vi "Config HW Set.vi"(6 "Send Cmd Timout(ms)":u32=300, 7 "CANcoder Ref":T1, 8 "Error":errorcluster, 9 "HW Config":T7={"ExtendHW Ver"=0, "CAN"={"ID"=0, "Bus"=""}, "Output"={"Type"=enum."Counter-Clockwise", "Neutral"=enum."EEPROMSetting", "Max"={"FWD"=0.0, "REV"=-1.0}, "Min"={"FWD"=0.0, "REV"=0.0}, "OL Ramp Rate (S)"=0.0, "Dead Band"=0.0, "CL Ramp Rate (S)"=0.0}, "CL"={"Gains"={"P"=1.0, "I"=0.01, "D"=0.0, "F"=0.0}, "Error Allowed"=0.0, "I Zone"=0.0, "Peak Out 0-1"=10000.0, "Max I Accu"=-1000.0}, "MM"={"Cruise Velocity"=5000, "Acceleration"=5000}, "TravelLimits"={"Hard"={"FWD Switch Normal"=enum."Normally Open", "FWD On will Zero Encoder "=FALSE, "REV Switch Normal"=enum."Normally Open", "REV On will Zero Encoder "=FALSE}, "Soft"={"FWD"={"Enable"=FALSE, "Counts"=0}, "REV"={"Enable"=FALSE, "Counts"=0}}}, "StatorLimit"={"Enable"=FALSE, "Current Limit"=0.0, "Threshold Current"=0.0, "Threshold Time"=0.0}, "Cancoder"={"ID"=0, "CW(t) CCW(f)"=TRUE, "Zero Offset"=0.0}} {"TravelLimits"."Soft"."REV"."Counts" format="%#.0f"; "TravelLimits"."Soft"."FWD"."Counts" format="%#.0f"; "Output"."Min"."REV" format="%.2f"; "Output"."Min"."FWD" format="%.2f"; "Output"."Max"."REV" format="%.2f"; "Output"."Max"."FWD" format="%.2f"; "CL"."Gains"."F" format="%#.8f"; "CL"."Gains"."D" format="%#.8f"; "CL"."Gains"."I" format="%#.8f"; "CL"."Gains"."P" format="%#.8f"}, 10 "Max # Of Tries":i32, 11 "DevRef":T2={"DeviceStatus"={"status"=FALSE, "code"=0, "source"=""}, "Type"=enum."PWM", "PWM"={"PWM Channel"=enum."Invalid", "DeadBand"={"Name"="", "maxPositivePwm"=0, "minPositivePwm"=0, "centerPwm"=0, "maxNegativePwm"=0, "minNegativePwm"=0, "angularRange"=0}}, "CAN"={"Device Number"=0, "SetOutput VI Ref"=variant, "GetOutput VI Ref"=variant, "Enable VI Ref"=variant, "Disable VI Ref"=variant, "Data"=variant}, "Invert"=FALSE, "DIO PWM"={"PWM \"Enable\" Channel"=enum."Invalid", "DIOChannel"=enum."Invalid", "PWM Rate"=0.0}}) -> (0 "Error Out":errorcluster, 3 "DevRef Out Out":T2, 5 "CANcoder Ref Out":T1)   [LabVIEW 2023, in "2024 AdPivotArm_ACT.lvlib"]
uses:
  2024 AdPivotArm_ACT.lvlib
  Shared Code/TypeDefs/Cluster_Extend_Config HW Values.ctl
  Shared Code/TypeDefs/Cluser_CAN Data.ctl
  Shared Code/TypeDefs/Cluster_Config FX Motor Output.ctl
  <vilib>/Rock Robotics/WPI/ThirdParty/Phoenix-LabVIEW/Motor Controller/Controls/CTRE_Phoenix_MotorControl_TalonFXInvertType.ctl
  <vilib>/Rock Robotics/WPI/ThirdParty/Phoenix-LabVIEW/Motor Controller/Controls/CTRE_Phoenix_MotorControl_NeutralMode.ctl
  Shared Code/TypeDefs/Cluster_FWD  REV Values.ctl
  Shared Code/TypeDefs/Cluster_FX SLOT PID Config.ctl
  Shared Code/TypeDefs/Cluster_PID Gains.ctl
  Shared Code/TypeDefs/Cluster_FX Motion Magic Parameters.ctl
  Shared Code/TypeDefs/Cluser_FX Config_Limit Travel.ctl
  Shared Code/TypeDefs/Cluser_Hard Limits.ctl
  <vilib>/Rock Robotics/WPI/ThirdParty/Phoenix-LabVIEW/Motor Controller/Controls/CTRE_Phoenix_MotorControl_LimitSwitchNormal.ctl
  Shared Code/TypeDefs/Cluser_Config_Soft Limits.ctl
  Shared Code/TypeDefs/Cluser_Enable-Value I32.ctl
  Shared Code/TypeDefs/Cluser_FX Config_Current Limits.ctl
  Shared Code/TypeDefs/Cluster_Cancoder_Config Data.ctl
  <vilib>/Rock Robotics/WPI/MotorControl/WPI_MotorControlDeviceRef.ctl
  <vilib>/Rock Robotics/WPI/MotorControl/WPI_MotorControlType.ctl
  <vilib>/Rock Robotics/SystemInterfaces/DIO/FPGA_DIOPWMChannel.ctl
  <vilib>/Rock Robotics/WPI/PWM/WPI_PWMDeadband.ctl
  <vilib>/Rock Robotics/SystemInterfaces/DIO/FPGA_DIOChannel.ctl
  <vilib>/Rock Robotics/WPI/ThirdParty/Phoenix-LabVIEW/CANCoder/Controls/CTRE_Phoenix_CANcoder_DeviceRef.ctl
  Shared Code/TypeDefs/Cluster_Config Motor Output.ctl
  Shared Code/TypeDefs/Cluster_PID Config.ctl
  Shared Code/TypeDefs/Cluster_High-Low.ctl
  Shared Code/TypeDefs/Cluster_Motion Magic Parameters.ctl
  Shared Code/TypeDefs/Cluster_Config_Cancoder Data.ctl
panel:
  # "Tune Output\nto 1023 Max"
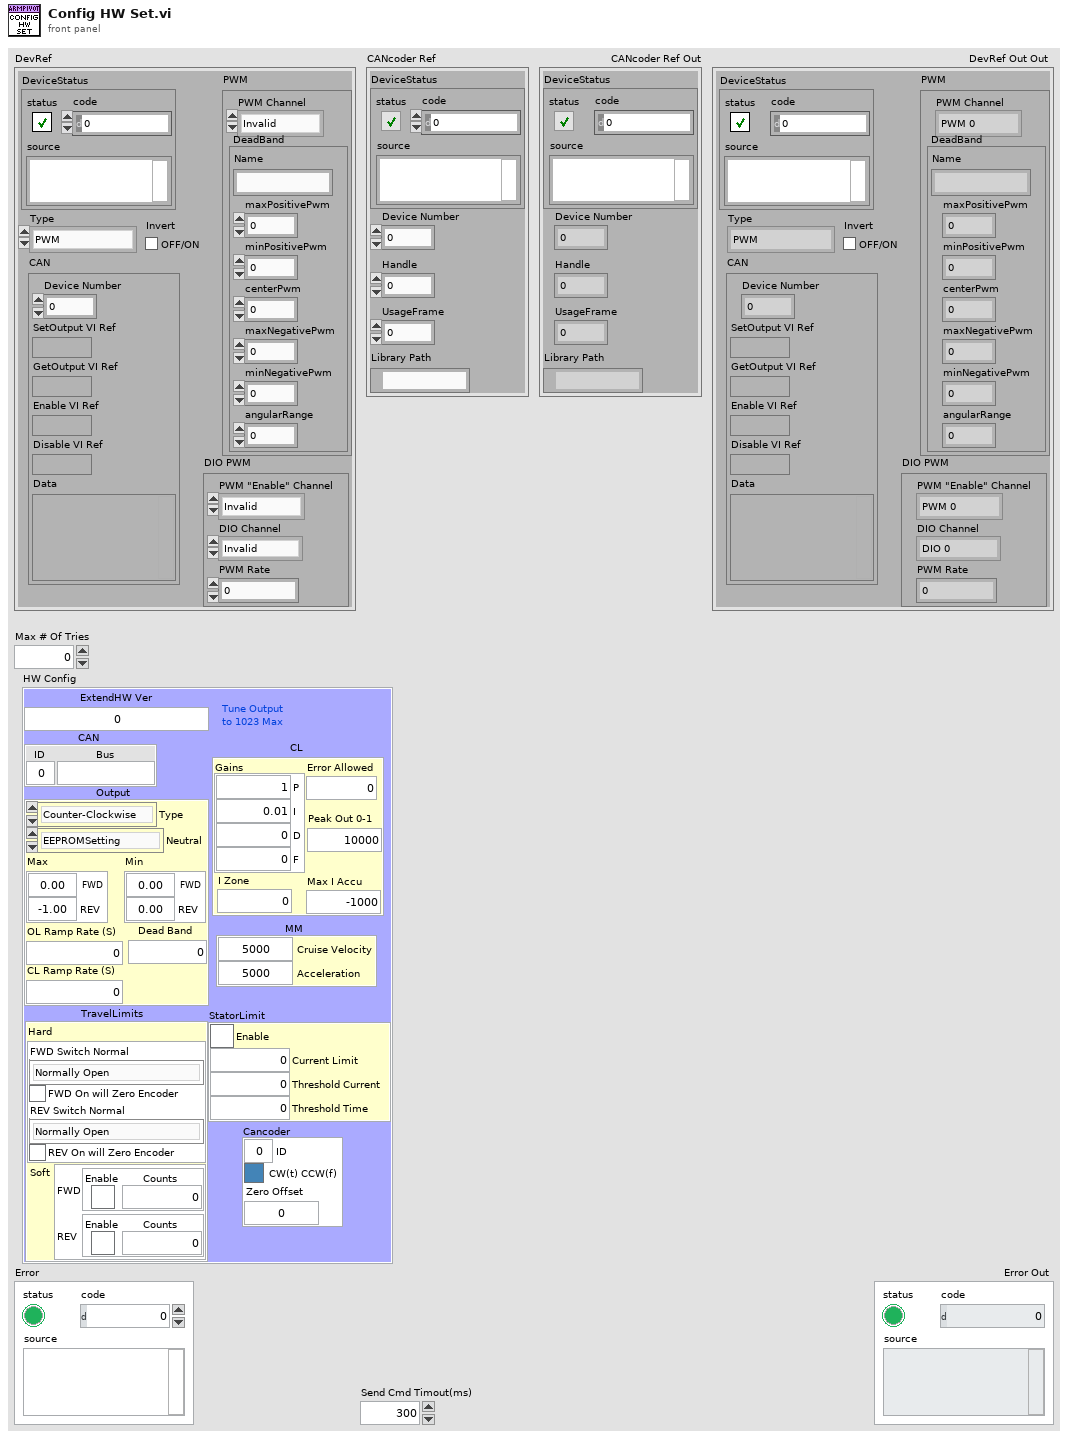
[diagram p1: front panel]
types:
  T1 = typedef "CTRE_Phoenix_CANcoder_DeviceRef.ctl" = cluster{"DeviceStatus":errorcluster, "Device Number":u8, "Handle":u64, "UsageFrame":u32, "Library Path":path}
  T2 = typedef "WPI_MotorControlDeviceRef.ctl" = cluster{"DeviceStatus":errorcluster, "Type":T3, "PWM":cluster{"PWM Channel":T4, "DeadBand":T5}, "CAN":cluster{"Device Number":u8, "SetOutput VI Ref":variant, "GetOutput VI Ref":variant, "Enable VI Ref":variant, "Disable VI Ref":variant, "Data":variant}, "Invert":bool, "DIO PWM":cluster{"PWM \"Enable\" Channel":T4, "DIOChannel":T6, "PWM Rate":dbl}}
  T3 = typedef "WPI_MotorControlType.ctl" = enum16{"PWM", "CAN", "DIO PWM"}
  T4 = typedef "FPGA_DIOPWMChannel.ctl" = enum8{"PWM 0", "PWM 1", "PWM 2", "PWM 3", "PWM 4", "PWM 5", "PWM 6", "PWM 7", "PWM 8", "PWM 9", "PWM MXP 0", "PWM MXP 1", "PWM MXP 2", "PWM MXP 3", "PWM MXP 4", "PWM MXP 5", "PWM MXP 6", "PWM MXP 7", "PWM MXP 8", "PWM MXP 9", "Invalid"}
  T5 = typedef "WPI_PWMDeadband.ctl" = cluster{"Name":string, "maxPositivePwm":i32, "minPositivePwm":i32, "centerPwm":i32, "maxNegativePwm":i32, "minNegativePwm":i32, "angularRange":u16}
  T6 = typedef "FPGA_DIOChannel.ctl" = enum8{"DIO 0", "DIO 1", "DIO 2", "DIO 3", "DIO 4", "DIO 5", "DIO 6", "DIO 7", "DIO 8", "DIO 9", "DIO MXP 0", "DIO MXP 1", "DIO MXP 2", "DIO MXP 3", "DIO MXP 4", "DIO MXP 5", "DIO MXP 6", "DIO MXP 7", "DIO MXP 8", "DIO MXP 9", "DIO MXP 10", "DIO MXP 11", "DIO MXP 12", "DIO MXP 13", "DIO MXP 14", "DIO MXP 15", "SPI Port CS1", "SPI Port CS2", "SPI Port CS3", "SPI Port MISO", "SPI Port MOSI", "Invalid"}
  T7 = typedef "Cluster_Extend_Config HW Values.ctl" = cluster{"ExtendHW Ver":u64, "CAN":T8, "Output":T9, "CL":T13, "MM":T15, "TravelLimits":T16, "StatorLimit":T21, "Cancoder":T22}
  T8 = typedef "Cluser_CAN Data.ctl" = cluster{"ID":u8, "Bus":string}
  T9 = typedef "Cluster_Config FX Motor Output.ctl" = cluster{"Type":T10, "Neutral":T11, "Max":T12, "Min":T12, "OL Ramp Rate (S)":dbl, "Dead Band":dbl, "CL Ramp Rate (S)":dbl}
  T10 = typedef "CTRE_Phoenix_MotorControl_TalonFXInvertType.ctl" = enum16{"Counter-Clockwise", "Clockwise"}
  T11 = typedef "CTRE_Phoenix_MotorControl_NeutralMode.ctl" = enum8{"EEPROMSetting", "Override to Coast", "Override to Brake"}
  T12 = typedef "Cluster_FWD  REV Values.ctl" = cluster{"FWD":dbl, "REV":dbl}
  T13 = typedef "Cluster_FX SLOT PID Config.ctl" = cluster{"Gains":T14, "Error Allowed":dbl, "I Zone":dbl, "Peak Out 0-1":dbl, "Max I Accu":dbl}
  T14 = typedef "Cluster_PID Gains.ctl" = cluster{"P":dbl, "I":dbl, "D":dbl, "F":dbl}
  T15 = typedef "Cluster_FX Motion Magic Parameters.ctl" = cluster{"Cruise Velocity":i32, "Acceleration":i32}
  T16 = typedef "Cluser_FX Config_Limit Travel.ctl" = cluster{"Hard":T17, "Soft":T19}
  T17 = typedef "Cluser_Hard Limits.ctl" = cluster{"FWD Switch Normal":T18, "FWD On will Zero Encoder ":bool, "REV Switch Normal":T18, "REV On will Zero Encoder ":bool}
  T18 = typedef "CTRE_Phoenix_MotorControl_LimitSwitchNormal.ctl" = enum16{"Normally Open", "Normally Closed", "Disabled"}
  T19 = typedef "Cluser_Config_Soft Limits.ctl" = cluster{"FWD":T20, "REV":T20}
  T20 = typedef "Cluser_Enable-Value I32.ctl" = cluster{"Enable":bool, "Counts":i32}
  T21 = typedef "Cluser_FX Config_Current Limits.ctl" = cluster{"Enable":bool, "Current Limit":dbl, "Threshold Current":dbl, "Threshold Time":dbl}
  T22 = typedef "Cluster_Cancoder_Config Data.ctl" = cluster{"ID":u8, "CW(t) CCW(f)":bool, "Zero Offset":dbl}
  T23 = typedef "Cluster_Config_Cancoder Data.ctl" = cluster{"ID":u8, "CW(t) CCW(f)":bool, "Zero Offset":dbl}
  T24 = typedef "Cluster_Motion Magic Parameters.ctl" = cluster{"Cruise Velocity":i32, "Acceleration":i32}
  T25 = typedef "Cluster_PID Config.ctl" = cluster{"Gains":T14, "Error Allowed":T26, "I Zone":T26, "Max Out":T12, "Max I Accu":T26, "CL Ramp Rate (S)":dbl}
  T26 = typedef "Cluster_High-Low.ctl" = cluster{"High":dbl, "Low":dbl}
  T27 = typedef "Cluster_Config Motor Output.ctl" = cluster{"Type":T10, "Neutral":T11, "Max":T12, "Min":T12, "OL Ramp Rate (S)":dbl, "Dead Band":dbl}
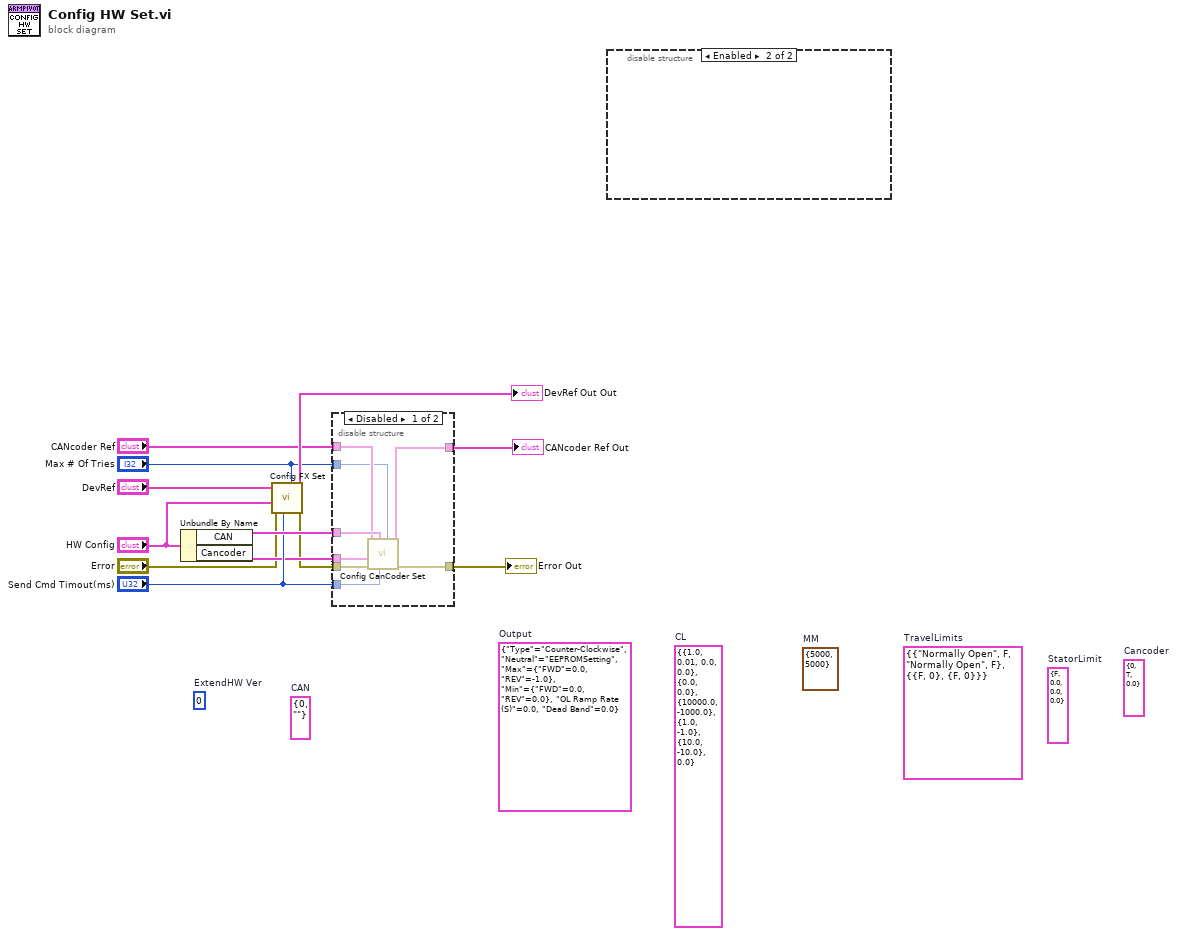
[diagram p0: block diagram]
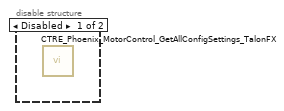
[diagram p3: hidden frame]
diagram:
  (unwired) T23 {"ID"=0, "CW(t) CCW(f)"=TRUE, "Zero Offset"=0.0}  # Cancoder
  (unwired) T21 {"Enable"=FALSE, "Current Limit"=0.0, "Threshold Current"=0.0, "Threshold Time"=0.0}  # StatorLimit
  (unwired) T24 {"Cruise Velocity"=5000, "Acceleration"=5000}  # MM
  (unwired) T16 {"Hard"={"FWD Switch Normal"=enum."Normally Open", "FWD On will Zero Encoder "=FALSE, "REV Switch Normal"=enum."Normally Open", "REV On will Zero Encoder "=FALSE}, "Soft"={"FWD"={"Enable"=FALSE, "Counts"=0}, "REV"={"Enable"=FALSE, "Counts"=0}}}  # TravelLimits
  (unwired) T25 {"Gains"={"P"=1.0, "I"=0.01, "D"=0.0, "F"=0.0}, "Error Allowed"={"High"=0.0, "Low"=0.0}, "I Zone"={"High"=10000.0, "Low"=-1000.0}, "Max Out"={"FWD"=1.0, "REV"=-1.0}, "Max I Accu"={"High"=10.0, "Low"=-10.0}, "CL Ramp Rate (S)"=0.0}  # CL
  (unwired) T27 {"Type"=enum."Counter-Clockwise", "Neutral"=enum."EEPROMSetting", "Max"={"FWD"=0.0, "REV"=-1.0}, "Min"={"FWD"=0.0, "REV"=0.0}, "OL Ramp Rate (S)"=0.0, "Dead Band"=0.0}  # Output
  (unwired) T8 {"ID"=0, "Bus"=""}  # CAN
  (unwired) u64 0  # ExtendHW Ver
  n1 = Unbundle By Name("HW Config") -> ("CAN"=w9:T8, "Cancoder"=w4:T22)
  n2 = call "Config FX Set.vi"("Max # Of Tries"="Max # Of Tries", "Send Cmd Timout(ms)"="Send Cmd Timout(ms)", "Error"="Error", "HW Config"="HW Config", "DevRef"="DevRef") -> ("Error Out"=w3:errorcluster, "DevRef Out Out"=→"DevRef Out Out":T2)  [unwired: 5 in]
  n3 = disable-structure shown="Disabled" {
    disable-tunnel: w9 -> [w20 _]
    disable-tunnel: "CANcoder Ref" -> [w19 w22]
    disable-tunnel: [w18 w22] -> w7
    disable-tunnel: "Max # Of Tries" -> [w17 _]
    disable-tunnel: "Send Cmd Timout(ms)" -> [w16 _]
    disable-tunnel: w4 -> [w15 _]
    disable-tunnel: w3 -> [w14 w21]
    disable-tunnel: [w13 w21] -> w1
    frame Disabled {
      n4 = call "Config CanCoder Set.vi"("Max # Of Tries"=w17, "Send Cmd Timout(ms)"=w16, "CAN"=w20, "Error"=w14, "Can Coder Data"=w15, "CANcoder Ref"=w19) -> ("Error Out"=w13:errorcluster, "CANcoder Ref Out"=w18:T1)  [unwired: 4 in]
    }
    frame Enabled {
    }
  }
  "Error Out" <- w1
  "CANcoder Ref Out" <- w7
  n5 = disable-structure shown="Enabled" {
    frame Disabled {
      n6 = call <vilib>:"CTRE_Phoenix_MotorControl_GetAllConfigSettings_TalonFX.vi"() -> ()  [unwired: 9 in, 3 out]
    }
    frame Enabled {
    }
  }
